vi "Simple Read.vi"(4 "Read":refnum<class "Abs_U8 Integer.lvclass">) -> (1 "Value":u8)   [LabVIEW 2021, in "Abs_U8 Integer.lvclass"]
uses:
  Abs_U8 Integer.lvclass
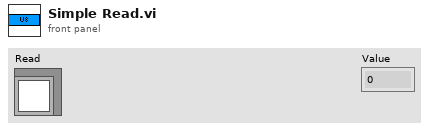
[diagram p1: front panel]
types:
  T1 = typedef "Abs_U8 Integer.lvclass/Type.ctl" = u8
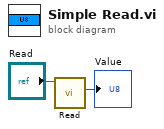
[diagram p0: block diagram]
diagram:
  n1 = call-dynamic "Read.vi"("Double Float.lvclass_340760 in"="Read") -> ("Value"=→"Value":T1)  [unwired: 8 in, 2 out]
